vi "Get Pressure Readings.vi"(8 "error in (no error)":errorcluster) -> (0 "error out":errorcluster, 2 "NI DAQ Leak Pressure":dbl, 3 "NI-DAQ Pressure":dbl, 5 "Oil Pressure":dbl)   [LabVIEW 2015]
uses:
  Common/Buffers/Snapshot/Snapshot.lvclass
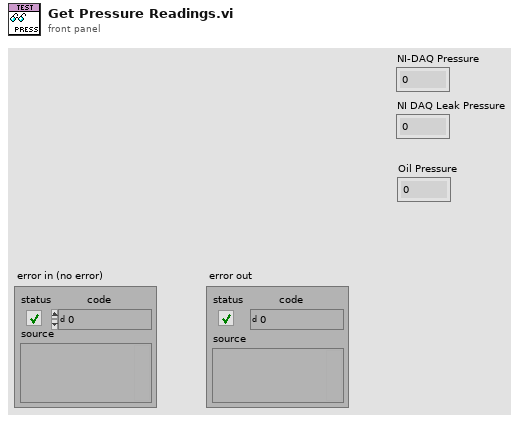
[diagram p1: front panel]
types:
  T1 = typedef "Snapshot.lvclass/Session Handle.ctl" = refnum<data-value>
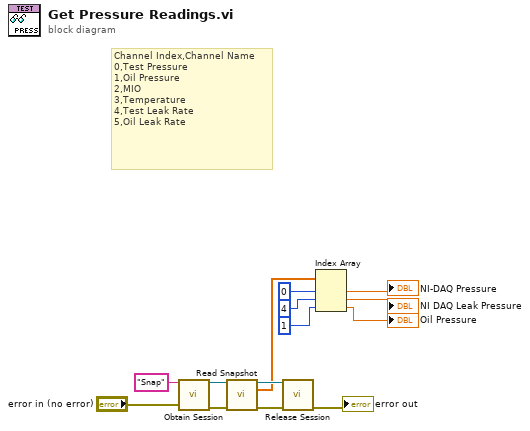
[diagram p0: block diagram]
diagram:
  # "Channel Index,Channel Name\n0,Test Pressure\n1,Oil Pressure\n2,MIO\n3,Temperature\n4,Test Leak Rate\n5,Oil Leak Rate"
  n1 = call "Obtain Session.vi"("Session  Name ()"="Snap", "error in (no error)"="error in (no error)") -> ("Session Handle"=w11:T1, "error out"=w12:errorcluster)  [unwired: 12 in]
  n2 = call "Read Snapshot.vi"("Session Handle in"=w11, "error in (no error)"=w12) -> ("Session Handle out"=w9:T1, "Buffer"=w7:dbl[], "error out"=w10:errorcluster)  [unwired: 11 in]
  n3 = call "Release Session.vi"("Session Handle"=w9, "error in (no error)"=w10) -> ("error out"=→"error out":errorcluster)  [unwired: 13 in]
  n4 = Index Array(array=w7, index #1=0 ("index"), index #2=4 ("index"), index #3=1 ("index")) -> (element #1=→"NI-DAQ Pressure":dbl, element #2=→"NI DAQ Leak Pressure":dbl, element #3=→"Oil Pressure":dbl)
